vi "HP_testbench_SCADA_application.vi"() -> ()   [LabVIEW 2025]
uses:
  <vilib>/addons/control/pid/NI_PID_pid.lvlib
  <vilib>/addons/control/pid/pid.llb/PID (DBL).vi
  <vilib>/express/express arith-compare/Formula/XNode/ExpressFormulaBlockNode.xnode
  <vilib>/Analysis/NI_AALBase.lvlib
  <vilib>/Analysis/baseanly.llb/Mean (DBL).vi
  <vilib>/express/express shared/transition.llb/Dynamic To Waveform Array.vi
  <vilib>/express/express arith-compare/Formula/Block/exnFormulaBlock how many pts in the wave.vi
  <vilib>/express/express shared/ex_Modify Signal Name.vi
  <vilib>/express/express shared/transition.llb/Waveform Array To Dynamic.vi
  <vilib>/express/express signal manip/GetorSetDDTAttributes/Get DDT Attributes/Get DDT Properties.xnode
  <vilib>/express/express signal manip/GetorSetDDTAttributes/Set DDT Attributes/Set DDT Properties.xnode
  <vilib>/express/express signal manip/GetorSetDDTAttributes/Set DDT Attributes/SetT0.vi
  <vilib>/express/express signal manip/GetorSetDDTAttributes/Set DDT Attributes/sub Set StartTimeStamp.vi
  <vilib>/express/express signal manip/GetorSetDDTAttributes/Set DDT Attributes/Set DDT Attributes.lvlib
  <vilib>/express/express signal manip/GetorSetDDTAttributes/Shared VIs/TimeType.ctl
  <vilib>/express/express signal manip/GetorSetDDTAttributes/Shared VIs/GetSetShared.lvlib
panel:
  in  "Start Local Data Backup":bool
  out "garbage_coll":dbl
  out "Numeric 2":i32
  out "Numeric":i32
  in  "Error when Server Start":errorcluster
  out "Internal Server Error":errorcluster
  out "Third Cycle Flowrate":dbl format="%0.2f"
  out "Heating Cycle Flowrate":dbl format="%0.2f"
  out "Cooling Cycle Flowrate":dbl format="%0.2f"
  out "Current":dbl format="%0.2f"
  out "Out H.E":dbl format="%0.2f"
  out "Out Aero":dbl format="%0.2f"
  out "In Froid":dbl format="%0.2f"
  out "Out Froid":dbl format="%0.2f"
  out "Out Chaud":dbl format="%0.2f"
  out "In Chaud":dbl format="%0.2f"
  out "current time":timestamp
  out "Amb Temp":dbl format="%0.2f"
  in  "?":bool
  in  "dt (s) tank":dbl=-1.0 format="%.3f"
  in  "Reinitiaize Aerotherme PID?":bool
  in  "Reinitialize Tank PID?":bool
  out "Tank Chart 2":T1(graph)
  out "Aerotherme Chart":T1(graph)
  in  "PID gains 2":T2={"proportional gain (Kc)"=1.0, "integral time (Ti, min)"=0.01, "derivative time (Td, min)"=0.0} {"derivative time (Td, min)" format="%.3f"; "integral time (Ti, min)" format="%.3f"; "proportional gain (Kc)" format="%.3f"}
  in  "setpoint in froid":dbl format="%.2f"
  in  "output range 2":cluster{"output high":dbl, "output low":dbl}={"output high"=100.0, "output low"=-100.0} {"output low" format="%.2f"; "output high" format="%.2f"}
  in  "PID gains":T2={"proportional gain (Kc)"=1.0, "integral time (Ti, min)"=0.01, "derivative time (Td, min)"=0.0} {"derivative time (Td, min)" format="%.3f"; "integral time (Ti, min)" format="%.3f"; "proportional gain (Kc)" format="%.3f"}
  in  "Setpoint In Chaud":dbl format="%.2f"
  in  "output range":cluster{"output high":dbl, "output low":dbl}={"output high"=100.0, "output low"=-100.0} {"output low" format="%.2f"; "output high" format="%.2f"}
  # "STOP Aquiring & Twinning"
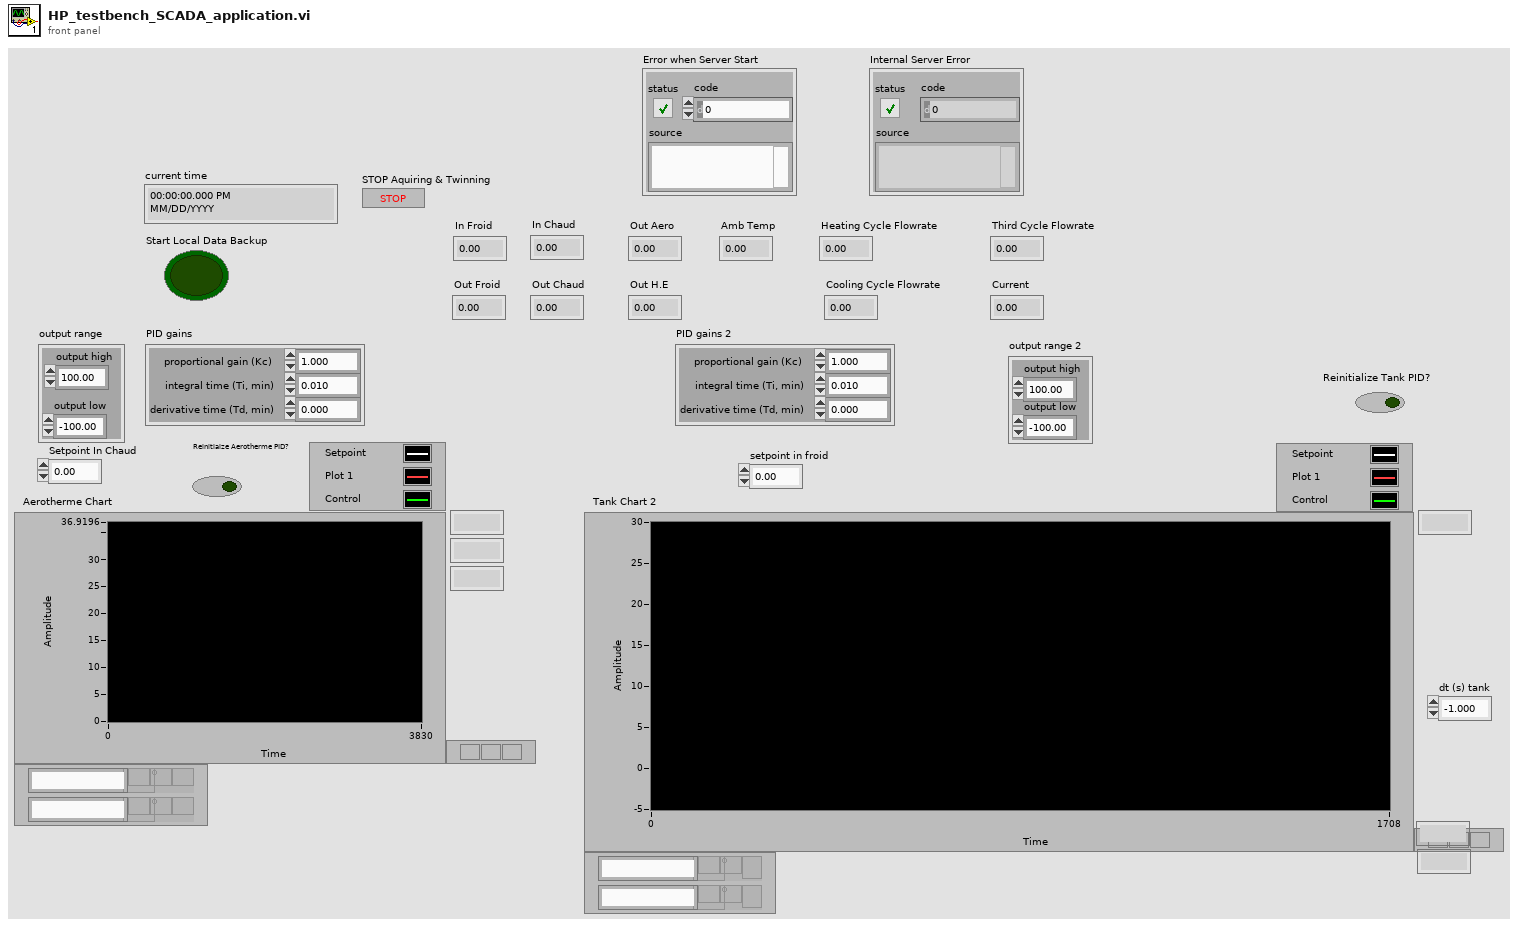
[diagram p1: front panel]
types:
  T1 = cluster{"Setpoint\n":dbl, "Plant Output":dbl, dbl}
  T2 = cluster{"proportional gain (Kc)":dbl, "integral time (Ti, min)":dbl, "derivative time (Td, min)":dbl}
  T3 = cluster{"Setpoint In Chaud":dbl, "mean":dbl, dbl}
  T4 = cluster{"setpoint in froid ":dbl, "mean":dbl, "output":dbl}
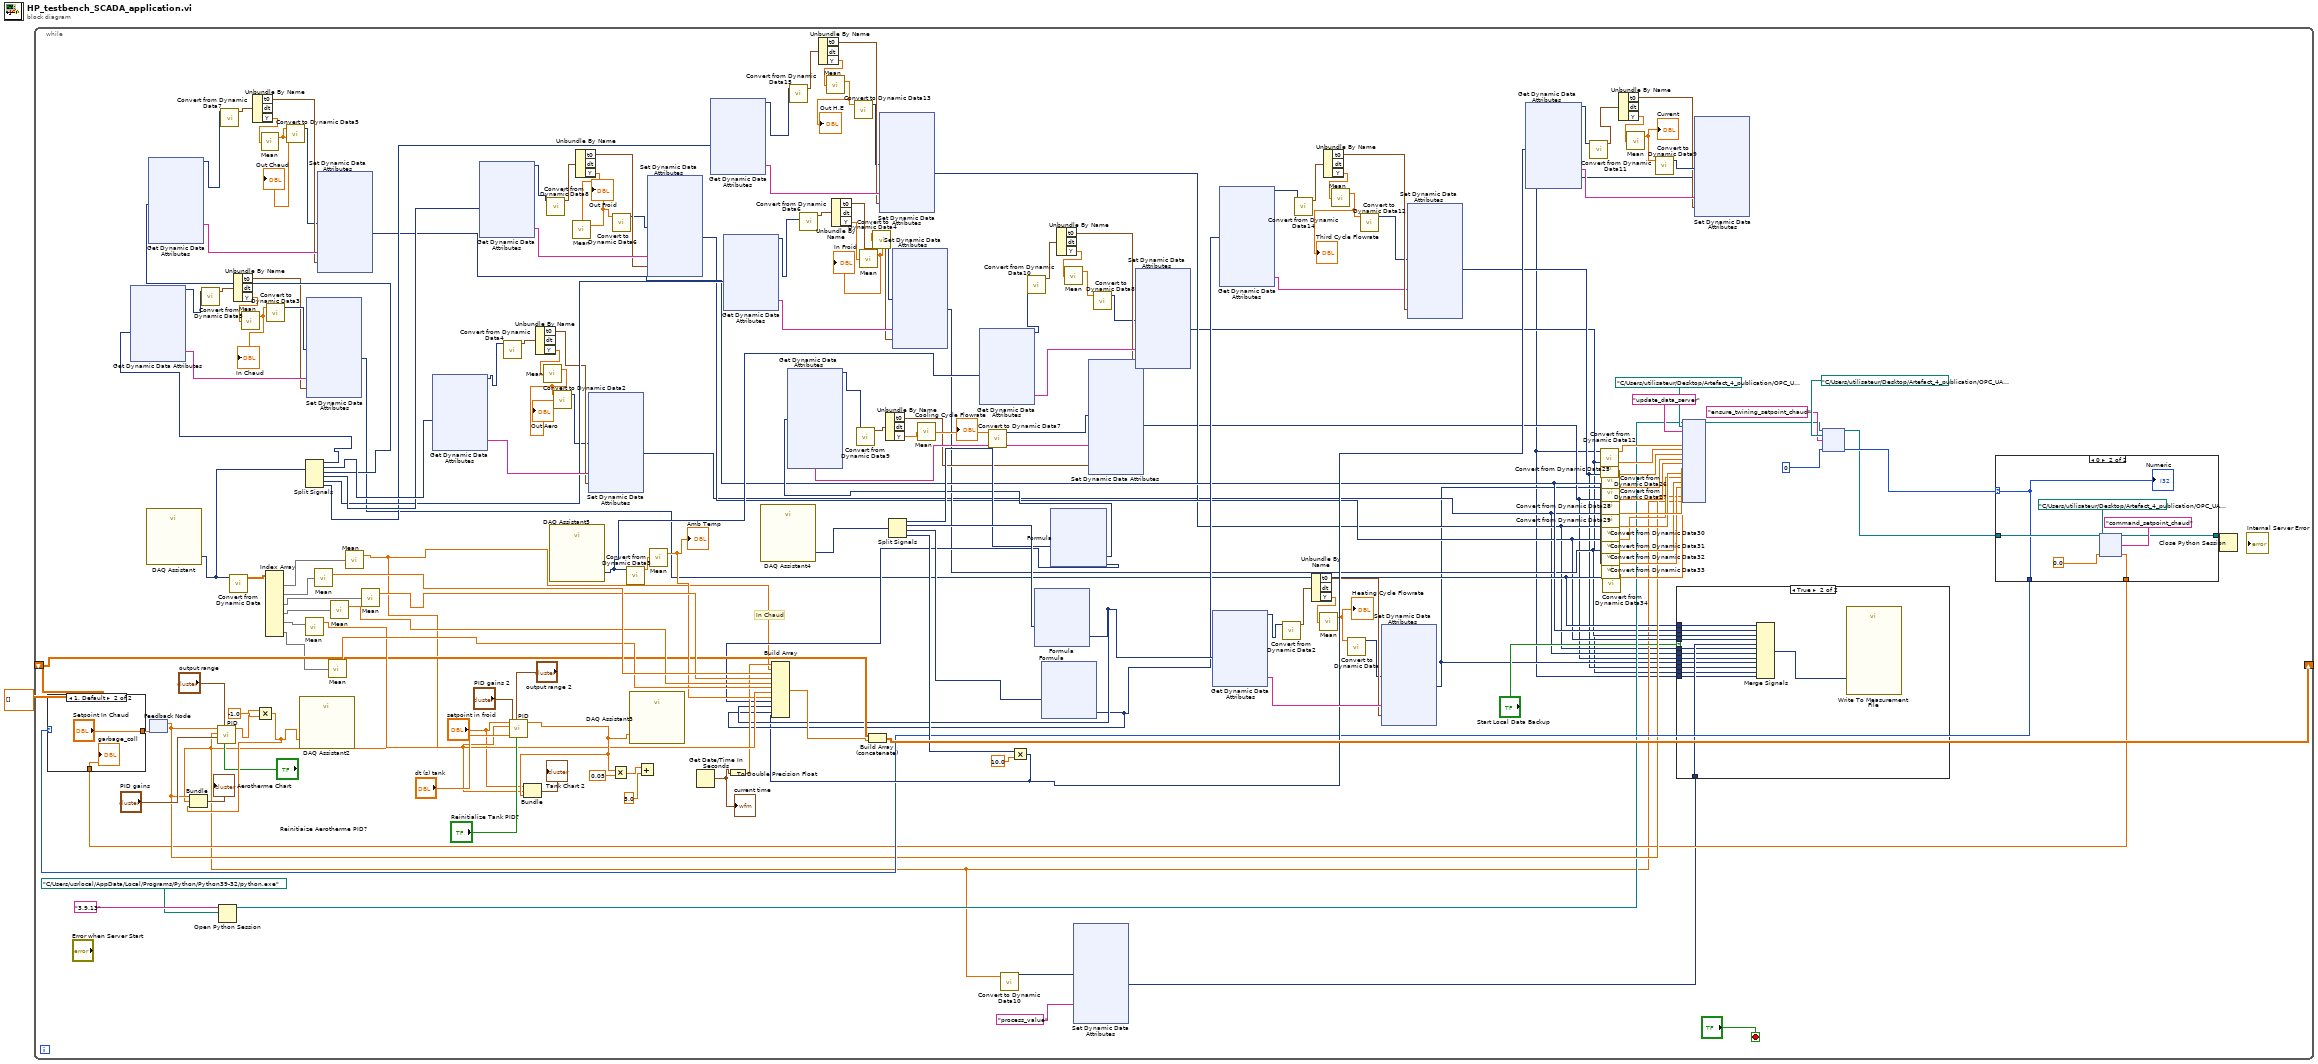
[diagram p0: block diagram]
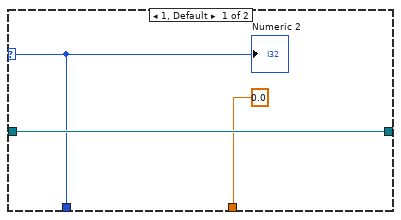
[diagram p4: hidden frame]
diagram:
  n1 = while {
    shift-right: [w144] -> _
    shift-left: dbl[][] [] -> [w143]
    stop <- "?" stop-if-true
    # "In Chaud"
    n2 = call "DAQ Assistant"() -> ("data"=w91:dynamicdata)  [unwired: 17 in, 2 out]
    n3 = feedback #1() -> (w24:dbl)  [unwired: 1 in]
    n4 = Open Python Session(python version="3.9.13" ("Python version"), python path=path "C:/Users/usrlocal/AppData/Local/Programs/Python/Python39-32/python.exe" ("Python path")) -> (session out=w18:refnum<k35>)  [unwired: 1 in, 1 out]
    n5 = call "Convert from Dynamic Data"("Dynamic Data Type"=w91) -> ("Array"=w176:dbl[][])  [unwired: 3 in]
    n6 = Index Array(array=w176) -> (element #1=w157:dbl[], element #2=w158:dbl[], element #3=w156:dbl[], element #4=w155:dbl[], element #5=w112:dbl[], element #6=w113:dbl[])  [unwired: 12 in]
    n7 = Split Signals(w91) -> (w136:dynamicdata, w131:dynamicdata, w130:dynamicdata, w129:dynamicdata, w126:dynamicdata, w114:dynamicdata)  [unwired: 6 in]
    n8 = xnode "Get Dynamic Data Attributes"("Signals In"=w136) -> ("Signal Name"=w135:string, "Signals Out"=w78:dynamicdata)  [unwired: 2 in, 1 out]
    n9 = xnode "Get Dynamic Data Attributes"("Signals In"=w130) -> ("Signal Name"=w134:string, "Signals Out"=w84:dynamicdata)  [unwired: 2 in, 2 out]
    n10 = call "Convert from Dynamic Data5"("Dynamic Data Type"=w78) -> ("Waveform"=w77:waveform(dbl))  [unwired: 3 in]
    n11 = call "Convert from Dynamic Data7"("Dynamic Data Type"=w84) -> ("Waveform"=w83:waveform(dbl))  [unwired: 3 in]
    n12 = Unbundle By Name(w77) -> ("t0"=w48:timestamp, "Y"=w75:dbl[])  [unwired: 1 out]
    n13 = call-poly <vilib>:"Mean.vi"("X"=w75) -> ("mean"=w74:dbl)  [unwired: 1 out]
    "In Chaud" <- w74
    n14 = Unbundle By Name(w83) -> ("t0"=w82:timestamp, "Y"=w81:dbl[])  [unwired: 1 out]
    n15 = call-poly <vilib>:"Mean.vi"("X"=w81) -> ("mean"=w79:dbl)  [unwired: 1 out]
    "Out Chaud" <- w79
    n16 = call "Convert to Dynamic Data3"("Double"=w74) -> ("Dynamic Data Type"=w76:dynamicdata)  [unwired: 3 in]
    n17 = call "Convert to Dynamic Data5"("Double"=w79) -> ("Dynamic Data Type"=w80:dynamicdata)  [unwired: 3 in]
    n18 = call-poly <vilib>:"Mean.vi"("X"=w112) -> ("mean"=w149:dbl)  [unwired: 1 out]
    n19 = xnode "Set Dynamic Data Attributes"("Signals In"=w76, "Signal Name"=w135, "Timestamp"=w48) -> ("Signals Out"=w16:dynamicdata)  [unwired: 2 in, 1 out]
    n20 = call-poly <vilib>:"Mean.vi"("X"=w158) -> ("mean"=w153:dbl)  [unwired: 1 out]
    n21 = xnode "Set Dynamic Data Attributes"("Signals In"=w80, "Signal Name"=w134, "Timestamp"=w82) -> ("Signals Out"=w15:dynamicdata)  [unwired: 2 in, 1 out]
    n22 = call-poly <vilib>:"Mean.vi"("X"=w113) -> ("mean"=w150:dbl)  [unwired: 1 out]
    n23 = call-poly <vilib>:"Mean.vi"("X"=w155) -> ("mean"=w151:dbl)  [unwired: 1 out]
    n24 = call-poly <vilib>:"Mean.vi"("X"=w157) -> ("mean"=w10:dbl)  [unwired: 1 out]
    n25 = call-poly <vilib>:"PID.vi"("reinitialize? (F)"="Reinitiaize Aerotherme PID?", "output range"="output range", "PID gains"="PID gains", "process variable"=w10, "setpoint"=w24) -> ("output"=w168:dbl)  [unwired: 5 in, 1 out]
    n26 = Multiply(x=w168, y=-1.0) -> (x*y=w160:dbl)
    n27 = Bundle("Setpoint In Chaud"=w24, "mean"=w10, w160) -> (→"Aerotherme Chart":T3)  [unwired: 1 in]
    n28 = call "DAQ Assistant2"("data"=w160) -> ()  [unwired: 17 in, 2 out]
    n29 = call-poly <vilib>:"Mean.vi"("X"=w156) -> ("mean"=w152:dbl)  [unwired: 1 out]
    n30 = xnode "Get Dynamic Data Attributes"("Signals In"=w131) -> ("Signal Name"=w133:string, "Signals Out"=w73:dynamicdata)  [unwired: 2 in, 1 out]
    n31 = xnode "Get Dynamic Data Attributes"("Signals In"=w129) -> ("Signal Name"=w132:string, "Signals Out"=w90:dynamicdata)  [unwired: 2 in, 1 out]
    n32 = call "Convert from Dynamic Data4"("Dynamic Data Type"=w73) -> ("Waveform"=w72:waveform(dbl))  [unwired: 3 in]
    n33 = call-poly <vilib>:"PID.vi"("reinitialize? (F)"="Reinitialize Tank PID?", "output range"="output range 2", "dt (s)"="dt (s) tank", "PID gains"="PID gains 2", "process variable"=w149, "setpoint"="setpoint in froid") -> ("output"=w161:dbl)  [unwired: 4 in, 1 out]
    n34 = Bundle("setpoint in froid"="setpoint in froid", "mean"=w149, "output"=w161) -> (→"Tank Chart 2":T4)  [unwired: 1 in]
    n35 = Unbundle By Name(w72) -> ("t0"=w71:timestamp, "Y"=w70:dbl[])  [unwired: 1 out]
    n36 = call-poly <vilib>:"Mean.vi"("X"=w70) -> ("mean"=w68:dbl)  [unwired: 1 out]
    "Out Aero" <- w68
    n37 = call "Convert from Dynamic Data8"("Dynamic Data Type"=w90) -> ("Waveform"=w89:waveform(dbl))  [unwired: 3 in]
    n38 = call "DAQ Assistant5"() -> ("data"=w115:dynamicdata)  [unwired: 17 in, 2 out]
    n39 = call "Convert to Dynamic Data2"("Double"=w68) -> ("Dynamic Data Type"=w69:dynamicdata)  [unwired: 3 in]
    n40 = Unbundle By Name(w89) -> ("t0"=w88:timestamp, "Y"=w87:dbl[])  [unwired: 1 out]
    n41 = call-poly <vilib>:"Mean.vi"("X"=w87) -> ("mean"=w85:dbl)  [unwired: 1 out]
    "Out Froid" <- w85
    n42 = xnode "Set Dynamic Data Attributes"("Signals In"=w69, "Signal Name"=w133, "Timestamp"=w71) -> ("Signals Out"=w7:dynamicdata)  [unwired: 2 in, 1 out]
    n43 = Multiply(x=w161, y=0.05) -> (x*y=w166:dbl)
    n44 = call "Convert to Dynamic Data6"("Double"=w85) -> ("Dynamic Data Type"=w86:dynamicdata)  [unwired: 3 in]
    n45 = call "Convert from Dynamic Data3"("Dynamic Data Type"=w115) -> ("Array"=w154:dbl[])  [unwired: 3 in]
    n46 = call "DAQ Assistant3"("data"=w161) -> ()  [unwired: 17 in, 2 out]
    n47 = Add(x=w166, y=5.0) -> ()  [unwired: 1 out]
    n48 = xnode "Set Dynamic Data Attributes"("Signals In"=w86, "Signal Name"=w132, "Timestamp"=w88) -> ("Signals Out"=w13:dynamicdata)  [unwired: 2 in, 1 out]
    n49 = call-poly <vilib>:"Mean.vi"("X"=w154) -> ("mean"=w148:dbl)  [unwired: 1 out]
    "Amb Temp" <- w148
    n50 = Get Date/Time In Seconds() -> (seconds since 1Jan1904=w147:timestamp)
    "current time" <- w147
    n51 = xnode "Get Dynamic Data Attributes"("Signals In"=w114) -> ("Signal Name"=w128:string, "Signals Out"=w102:dynamicdata)  [unwired: 2 in, 1 out]
    n52 = xnode "Get Dynamic Data Attributes"("Signals In"=w126) -> ("Signal Name"=w127:string, "Signals Out"=w67:dynamicdata)  [unwired: 2 in, 1 out]
    n53 = To Double Precision Float(number=w147) -> (double precision float=w146:dbl)
    n54 = call "DAQ Assistant4"() -> ("data"=w142:dynamicdata)  [unwired: 17 in, 2 out]
    n55 = call "Convert from Dynamic Data15"("Dynamic Data Type"=w102) -> ("Waveform"=w101:waveform(dbl))  [unwired: 3 in]
    n56 = call "Convert from Dynamic Data6"("Dynamic Data Type"=w67) -> ("Waveform"=w66:waveform(dbl))  [unwired: 3 in]
    n57 = Unbundle By Name(w101) -> ("t0"=w100:timestamp, "Y"=w99:dbl[])  [unwired: 1 out]
    n58 = call-poly <vilib>:"Mean.vi"("X"=w99) -> ("mean"=w50:dbl)  [unwired: 1 out]
    "Out H.E" <- w50
    n59 = Unbundle By Name(w66) -> ("t0"=w49:timestamp, "Y"=w65:dbl[])  [unwired: 1 out]
    n60 = call "Convert to Dynamic Data13"("Double"=w50) -> ("Dynamic Data Type"=w98:dynamicdata)  [unwired: 3 in]
    n61 = call-poly <vilib>:"Mean.vi"("X"=w65) -> ("mean"=w63:dbl)  [unwired: 1 out]
    "In Froid" <- w63
    n62 = call "Convert to Dynamic Data4"("Double"=w63) -> ("Dynamic Data Type"=w64:dynamicdata)  [unwired: 3 in]
    n63 = xnode "Set Dynamic Data Attributes"("Signals In"=w98, "Signal Name"=w128, "Timestamp"=w100) -> ("Signals Out"=w8:dynamicdata)  [unwired: 2 in, 1 out]
    n64 = Split Signals(w142) -> (w138:dynamicdata, w141:dynamicdata, w140:dynamicdata, w139:dynamicdata)  [unwired: 4 in]
    n65 = xnode "Set Dynamic Data Attributes"("Signals In"=w64, "Signal Name"=w127, "Timestamp"=w49) -> ("Signals Out"=w14:dynamicdata)  [unwired: 2 in, 1 out]
    n66 = xnode "Get Dynamic Data Attributes"("Signals In"=w115) -> ("Signal Name"=w116:string, "Signals Out"=w92:dynamicdata)  [unwired: 2 in, 1 out]
    n67 = call "Convert to Dynamic Data10"("Double"=w10) -> ("Dynamic Data Type"=w11:dynamicdata)  [unwired: 3 in]
    n68 = Multiply(x=w139, y=10.0) -> (x*y=w117:dynamicdata)
    n69 = call "Convert from Dynamic Data10"("Dynamic Data Type"=w92) -> ("Waveform"=w97:waveform(dbl))  [unwired: 3 in]
    n70 = xnode "Formula"("X1"=w141) -> ("Result"=w119:dynamicdata)  [unwired: 1 in, 1 out]
    n71 = xnode "Formula"("X1"=w140) -> ("Result"=w118:dynamicdata)  [unwired: 1 in, 1 out]
    n72 = xnode "Formula"("X1"=w138) -> ("Result"=w121:dynamicdata)  [unwired: 1 in, 1 out]
    n73 = Build Array(w146, w10, w153, w152, w151, w150, w149, w148, w121, w119, w118, w117) -> (w145:dbl[])
    n74 = xnode "Get Dynamic Data Attributes"("Signals In"=w121) -> ("Signal Name"=w137:string, "Signals Out"=w62:dynamicdata)  [unwired: 2 in, 3 out]
    n75 = call "Convert from Dynamic Data9"("Dynamic Data Type"=w62) -> ("Waveform"=w61:waveform(dbl))  [unwired: 3 in]
    n76 = Build Array (concatenate)(w143, w145) -> (w144:dbl[][])
    n77 = Unbundle By Name(w61) -> ("t0"=w57:timestamp, "Y"=w60:dbl[])  [unwired: 1 out]
    n78 = call-poly <vilib>:"Mean.vi"("X"=w60) -> ("mean"=w59:dbl)  [unwired: 1 out]
    "Cooling Cycle Flowrate" <- w59
    n79 = call "Convert to Dynamic Data7"("Double"=w59) -> ("Dynamic Data Type"=w58:dynamicdata)  [unwired: 3 in]
    n80 = Unbundle By Name(w97) -> ("t0"=w96:timestamp, "Y"=w95:dbl[])  [unwired: 1 out]
    n81 = call-poly <vilib>:"Mean.vi"("X"=w95) -> ("mean"=w94:dbl)  [unwired: 1 out]
    n82 = xnode "Set Dynamic Data Attributes"("Signals In"=w11, "Signal Name"="process_value") -> ("Signals Out"=w9:dynamicdata)  [unwired: 3 in, 1 out]
    n83 = xnode "Set Dynamic Data Attributes"("Signals In"=w58, "Signal Name"=w137, "Timestamp"=w57) -> ("Signals Out"=w6:dynamicdata)  [unwired: 3 in, 1 out]
    n84 = call "Convert to Dynamic Data8"("Double"=w94) -> ("Dynamic Data Type"=w93:dynamicdata)  [unwired: 3 in]
    n85 = xnode "Set Dynamic Data Attributes"("Signals In"=w93, "Signal Name"=w116, "Timestamp"=w96) -> ("Signals Out"=w3:dynamicdata)  [unwired: 2 in, 1 out]
    n86 = xnode "Get Dynamic Data Attributes"("Signals In"=w119) -> ("Signal Name"=w120:string, "Signals Out"=w56:dynamicdata)  [unwired: 2 in, 1 out]
    n87 = xnode "Get Dynamic Data Attributes"("Signals In"=w118) -> ("Signal Name"=w47:string, "Signals Out"=w107:dynamicdata)  [unwired: 2 in, 3 out]
    n88 = call "Convert from Dynamic Data2"("Dynamic Data Type"=w56) -> ("Waveform"=w55:waveform(dbl))  [unwired: 3 in]
    n89 = call "Convert from Dynamic Data14"("Dynamic Data Type"=w107) -> ("Waveform"=w106:waveform(dbl))  [unwired: 3 in]
    n90 = Unbundle By Name(w55) -> ("t0"=w54:timestamp, "Y"=w51:dbl[])  [unwired: 1 out]
    n91 = call-poly <vilib>:"Mean.vi"("X"=w51) -> ("mean"=w52:dbl)  [unwired: 1 out]
    "Heating Cycle Flowrate" <- w52
    n92 = Unbundle By Name(w106) -> ("t0"=w104:timestamp, "Y"=w105:dbl[])  [unwired: 1 out]
    n93 = call-poly <vilib>:"Mean.vi"("X"=w105) -> ("mean"=w108:dbl)  [unwired: 1 out]
    "Third Cycle Flowrate" <- w108
    n94 = call "Convert to Dynamic Data"("Double"=w52) -> ("Dynamic Data Type"=w53:dynamicdata)  [unwired: 3 in]
    n95 = call "Convert to Dynamic Data12"("Double"=w108) -> ("Dynamic Data Type"=w103:dynamicdata)  [unwired: 3 in]
    n96 = xnode "Set Dynamic Data Attributes"("Signals In"=w53, "Signal Name"=w120, "Timestamp"=w54) -> ("Signals Out"=w5:dynamicdata)  [unwired: 2 in, 1 out]
    n97 = xnode "Set Dynamic Data Attributes"("Signals In"=w103, "Signal Name"=w47, "Timestamp"=w104) -> ("Signals Out"=w4:dynamicdata)  [unwired: 3 in, 1 out]
    n98 = xnode "Get Dynamic Data Attributes"("Signals In"=w117) -> ("Signal Name"=w122:string, "Signals Out"=w123:dynamicdata)  [unwired: 2 in, 2 out]
    n99 = call "Convert from Dynamic Data11"("Dynamic Data Type"=w123) -> ("Waveform"=w111:waveform(dbl))  [unwired: 3 in]
    n100 = call "Convert from Dynamic Data25"("Dynamic Data Type"=w3) -> ("Scalar"=w45:dbl)  [unwired: 3 in]
    n101 = call "Convert from Dynamic Data26"("Dynamic Data Type"=w4) -> ("Scalar"=w44:dbl)  [unwired: 3 in]
    n102 = call "Convert from Dynamic Data27"("Dynamic Data Type"=w5) -> ("Scalar"=w43:dbl)  [unwired: 3 in]
    n103 = call "Convert from Dynamic Data28"("Dynamic Data Type"=w6) -> ("Scalar"=w42:dbl)  [unwired: 3 in]
    n104 = call "Convert from Dynamic Data29"("Dynamic Data Type"=w7) -> ("Scalar"=w41:dbl)  [unwired: 3 in]
    n105 = call "Convert from Dynamic Data30"("Dynamic Data Type"=w8) -> ("Scalar"=w40:dbl)  [unwired: 3 in]
    n106 = call "Convert from Dynamic Data31"("Dynamic Data Type"=w13) -> ("Scalar"=w39:dbl)  [unwired: 3 in]
    n107 = call "Convert from Dynamic Data32"("Dynamic Data Type"=w14) -> ("Scalar"=w38:dbl)  [unwired: 3 in]
    n108 = call "Convert from Dynamic Data33"("Dynamic Data Type"=w15) -> ("Scalar"=w37:dbl)  [unwired: 3 in]
    n109 = call "Convert from Dynamic Data34"("Dynamic Data Type"=w16) -> ("Scalar"=w36:dbl)  [unwired: 3 in]
    n110 = Unbundle By Name(w111) -> ("t0"=w109:timestamp, "Y"=w110:dbl[])  [unwired: 1 out]
    n111 = call-poly <vilib>:"Mean.vi"("X"=w110) -> ("mean"=w124:dbl)  [unwired: 1 out]
    "Current" <- w124
    n112 = call "Convert to Dynamic Data9"("Double"=w124) -> ("Dynamic Data Type"=w125:dynamicdata)  [unwired: 3 in]
    n113 = xnode "Set Dynamic Data Attributes"("Signals In"=w125, "Signal Name"=w122, "Timestamp"=w109) -> ("Signals Out"=w2:dynamicdata)  [unwired: 2 in, 1 out]
    n114 = call "Convert from Dynamic Data12"("Dynamic Data Type"=w2) -> ("Scalar"=w46:dbl)  [unwired: 3 in]
    n115 = case shown="True" "Start Local Data Backup" {
      tunnel: w16 -> [_ w206]
      tunnel: w15 -> [_ w205]
      tunnel: w14 -> [_ w204]
      tunnel: w13 -> [_ w203]
      tunnel: w9 -> [_ w202]
      tunnel: w8 -> [_ w201]
      tunnel: w7 -> [_ w200]
      tunnel: w6 -> [_ w199]
      tunnel: w5 -> [_ w198]
      tunnel: w4 -> [_ w197]
      tunnel: w3 -> [_ w196]
      tunnel: w2 -> [_ w195]
      frame False {
      }
      frame True {
        n116 = Merge Signals(w206, w205, w204, w203, w202, w201, w200, w199, w198, w197, w196, w195) -> (w207:dynamicdata)
        n117 = call "Write To Measurement File"("Signals"=w207) -> ()  [unwired: 16 in, 3 out]
      }
    }
    n118 = node(w18, path "C:/Users/utilisateur/Desktop/Artefact_4_publication/OPC_UA_DT_Server_Simulator.py" ("module path"), "update_data_server" ("function name"), w46, w45, w44, w43, w42, w41, w40, w39, w38, w37, w36, w24, w10) -> (w19:refnum<k35>)  [unwired: 16 in, 3 out]
    n119 = node(w19, path "C:/Users/utilisateur/Desktop/Artefact_4_publication/OPC_UA_DT_Server_Simulator.py" ("module path"), "ensure_twining_setpoint_chaud" ("function name"), 0) -> (w28:refnum<k35>, w29:i32)  [unwired: 1 in, 3 out]
    n120 = case shown="0" w29 {
      selector: w29 -> [w212 w214]
      tunnel: w28 -> [w213 w217]
      tunnel: [w213 w216] -> w22
      tunnel: [w212 w214] -> w26
      tunnel: [0.0 w215] -> w23
      frame 1, Default {
        "Numeric 2" <- w212
      }
      frame 0 {
        n121 = node(w217, path "C:/Users/utilisateur/Desktop/Artefact_4_publication/OPC_UA_DT_Server_Simulator.py" ("module path"), "command_setpoint_chaud" ("function name"), 0.0) -> (w216:refnum<k35>, w215:dbl)  [unwired: 1 in, 3 out]
        "Numeric" <- w214
      }
    }
    n122 = case shown="1, Default" w26 {
      tunnel: [w208 "Setpoint In Chaud"] -> w25
      tunnel: w23 -> [w208 w209]
      frame 0 {
      }
      frame 1, Default {
        "garbage_coll" <- w209
      }
    }
    n123 = feedback-in #1(w25) -> ()
    n124 = Close Python Session(session in=w22) -> ()  [unwired: 1 in, 1 out]
  }
